vi "ParseTxtFile.vi"(8 "error in":errorcluster, 11 "file path (use dialog)":path) -> (0 "error out":errorcluster, 2 "found?":bool, 3 "Commands Sent To SSM":string[](array[string])=["AcPwrInit", "AcPwrConfig", "AcPwrStartMeas,PPS,1", "AcPwrStartMeas,Chroma", "AcPwrDeviceOn,Chroma", "Delay,2000", "AcPwrDeviceOff,Chroma", "Delay,2000", "AcPwrDeviceOn,Chroma", "Delay,2000", "AcPwrDeviceOff,Chroma", "Delay,2000", "AcPwrDeviceOn,PPS", "AcPwrDeviceOff,PPS", "AcPwrClose,PPS", "AcPwrClose,Chroma", "Stop"])   [LabVIEW 2018, in "Test.lvclass"]
doc: "This VI reads a string of text commands from a provided text file and transforms the string into an array of commands. Each array entry is a command and the text file should be written such that a delimiter appears between each command. The default delimiters is an end of line. If a portion of the text file needs to be repeated ecase it in Loop and EndLoop for example:\n\nLoop\n\"Commands To Loop\"\nEndLoop"
uses:
  Test.lvclass
  <vilib>/Utility/config.llb/NI_LVConfig.lvlib
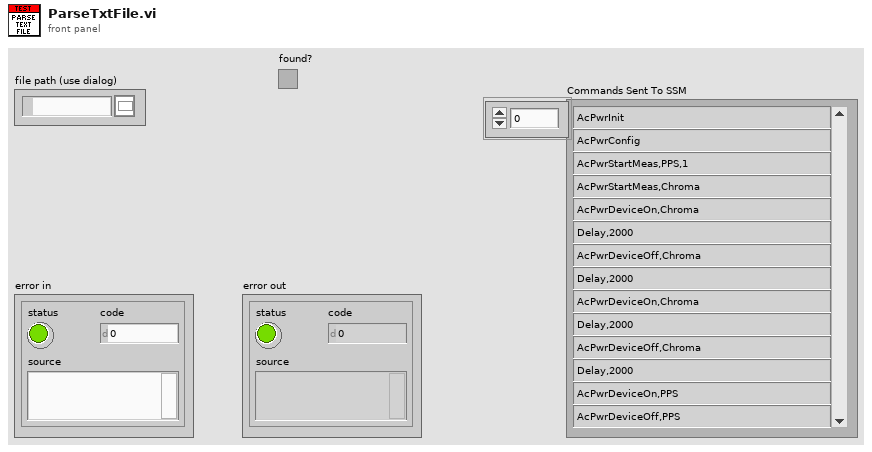
[diagram p1: front panel]
types:
  T1 = typedef "NI_LVConfig.lvlib/Config Data RefNum.ctl" = refnum<k1>
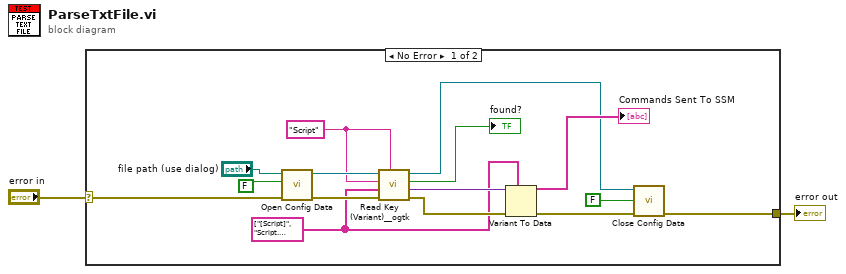
[diagram p0: block diagram]
diagram:
  n1 = case shown="No Error" "error in" {
    selector: "error in" -> [w10 w18]
    tunnel: [w3 w18] -> w1
    frame No Error {
      w8 = string[] ["[Script]", "Script.<size(s)> = \"7\"", "Script 0 = \"ErrorSeverity,Abort\"", "Script 1 = \"SensorCreateSession,SiemensDEM0\"", "Script 2 = \"SensorConfig,SiemensDEM0\"", "Script 3 = \"SensorStart,SiemensDEM0\"", "Script 4 = \"Delay,5000\"", "Script 5 = \"SensorStop,SiemensDEM0\""] ("Commands Sent To SSM")
      w12 = "Script" ("section")
      n2 = call <vilib>:"Open Config Data.vi"("error in (no error)"=w10, "create file if necessary (T)"=FALSE, "configuration file path"="file path (use dialog)") -> ("error out"=w15:errorcluster, "refnum"=w16:T1)  [unwired: 6 in, 1 out]
      n3 = call <userlib>:"Read Key (Variant)__ogtk.vi"("section"=w12, "error in (no error)"=w15, "type"=w8, "key (optional)"=w12, "refnum"=w16) -> ("error out"=w13:errorcluster, "key-value"=w14:variant, "found?"=→"found?":bool, "refnum out"=w4:T1)  [unwired: 3 in]
      n4 = Variant To Data(error in=w13, type=w8, Variant=w14) -> (data=→"Commands Sent To SSM":string[], error out=w5:errorcluster)
      n5 = call <vilib>:"Close Config Data.vi"("error in (no error)"=w5, "write file if changed (T)"=FALSE, "refnum"=w4) -> ("error out"=w3:errorcluster)  [unwired: 7 in, 1 out]
    }
    frame Error {
    }
  }
  "error out" <- w1
